vi "Save Workbook To File.vi"(8 "error in (no error)":errorcluster, 10 "File Name":path, 11 "Workbook Reference":refnum<k24>) -> (0 "error out":errorcluster, 3 "Workbook Reference Out":refnum<k24>)   [LabVIEW 2013]
uses:
  C:/PhaeronGit/LVNPOI/Resources/NPOI 2.1.1 dotnet2/NPOI.dll
  Resources/NPOI 2.1.1 dotnet2/NPOI.dll
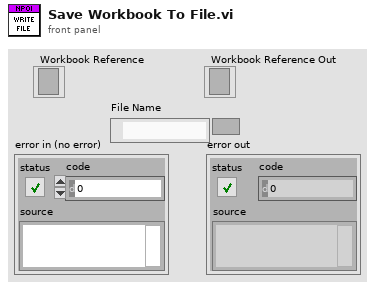
[diagram p1: front panel]
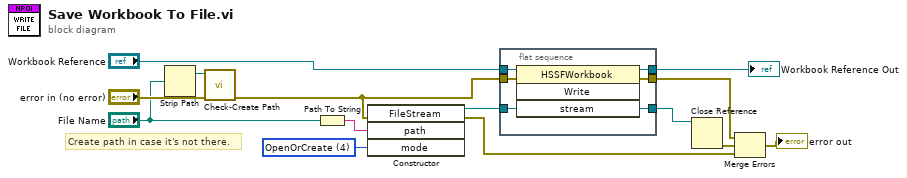
[diagram p0: block diagram]
diagram:
  w13 = 4 items=["CreateNew"=1, "Create"=2, "Open"=3, "OpenOrCreate"=4, "Truncate"=5, "Append"=6] ("mode")
  # "Create path in case it's not there."
  n1 = Strip Path(path="File Name") -> (stripped path=w1:path)  [unwired: 1 out]
  n2 = call <vilib>:"Check-Create Path.vi"("error in"="error in (no error)", "Path"=w1) -> ("error out"=w3:errorcluster)  [unwired: 8 in, 1 out]
  n3 = Path To String(path="File Name") -> (string=w14:string)
  n4 = constructor class="FileStream"(error in=w3, "path"=w14, "mode"=w13) -> (reference out=w10:refnum<k24>, error out=w5:errorcluster)  [unwired: 2 in, 3 out]
  n5 = flat-sequence {
    tunnel: "Workbook Reference" -> [w19]
    tunnel: [w18] -> w11
    tunnel: w3 -> [w17]
    tunnel: w10 -> [w15]
    tunnel: [w16] -> w9
    tunnel: [w15] -> w6
    frame #0 {
      n6 = invoke class="HSSFWorkbook" method="Write"(reference=w19, error in=w17, "stream"=w15) -> (reference out=w18:refnum<k24>, error out=w16:errorcluster)  [unwired: 1 in, 2 out]
    }
  }
  n7 = Close Reference(reference=w6) -> (error out=w7:errorcluster)  [unwired: 1 in]
  n8 = Merge Errors(w9, w7, w5) -> (→"error out":errorcluster)
  "Workbook Reference Out" <- w11
